vi "refreshRunFolder.vi"(8 "error in (no error)":errorcluster, 11 "Compiler in":refnum<class "Compiler.lvclass">) -> (0 "error out":errorcluster, 3 "Compiler out":refnum<class "Compiler.lvclass">)   [LabVIEW 2009, in "Compiler.lvlib" / "Compiler.lvclass"]
uses:
  Compiler.lvclass
  Compiler.lvclass/Compiler.ctl
  Filing/FileSystem/FileSystem.lvclass
panel:
  # "database has changed\nso all scripts should be\nrecompiled"
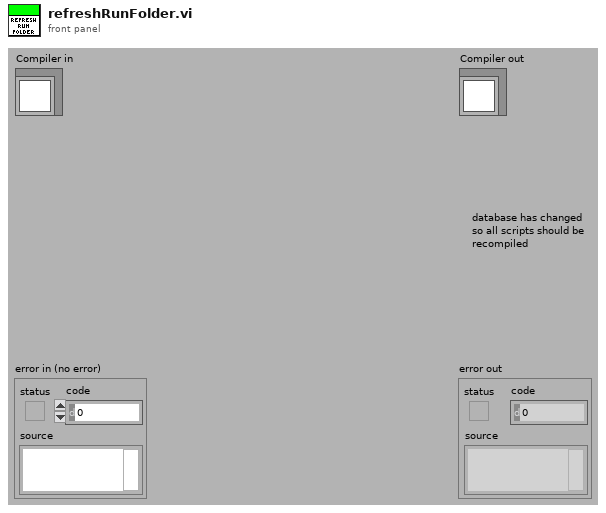
[diagram p1: front panel]
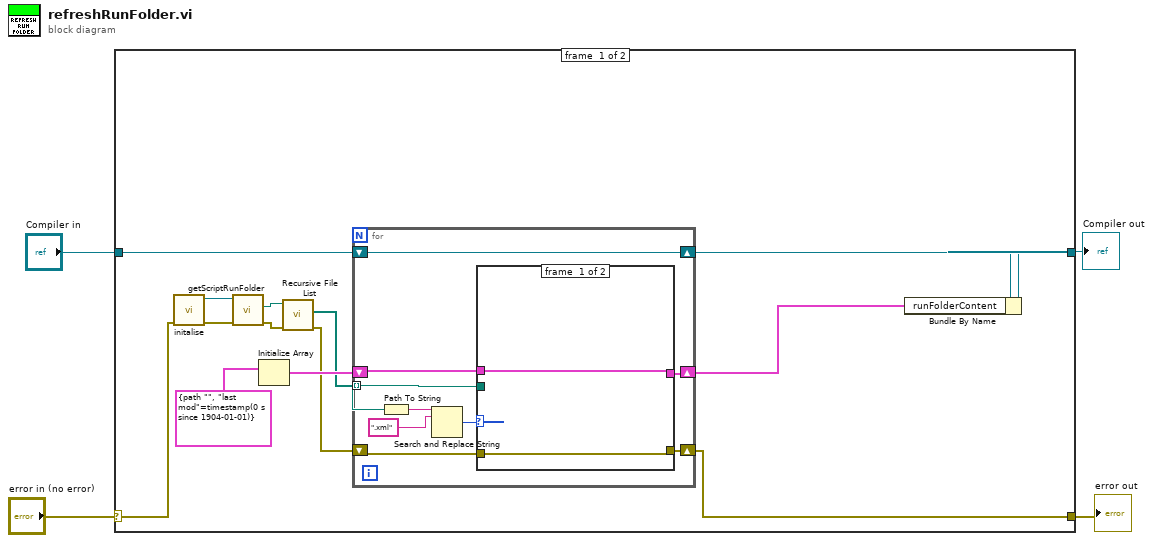
[diagram p0: block diagram]
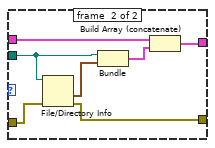
[diagram p2: hidden frame]
diagram:
  n1 = case shown="No Error" "error in (no error)" {
    selector: "error in (no error)" -> [w14 w38]
    tunnel: [w5 w38] -> w3
    tunnel: [w11 w37] -> w1
    tunnel: "Compiler in" -> [w9 w37]
    frame #0 {
      n2 = call "initalise.vi"("error in (no error)"=w14) -> ("error out"=w17:errorcluster, "FileSystem out"=w18:refnum<class "FileSystem.lvclass">)  [unwired: 9 in]
      n3 = call "getScriptRunFolder.vi"("error in (no error)"=w17, "FileSystem.lvclass in"=w18) -> ("error out"=w10:errorcluster, "ScriptRunFolder"=w16:path)  [unwired: 7 in, 1 out]
      n4 = Initialize Array(cluster{path, "last mod":timestamp} {path "", "last mod"=timestamp(0 s since 1904-01-01)} ("output cluster")) -> (w15:cluster{path, "last mod":timestamp}[])  [unwired: 1 in]
      n5 = call <vilib>:"Recursive File List.vi"("error in (no error)"=w10, "Folder Path"=w16) -> ("error out"=w6:errorcluster, "All Files in Dir"=w7:path[])  [unwired: 5 in, 3 out]
      n6 = for {
        tunnel: w7 -> [w23] mode=indexing
        shift-right: [w22] -> w8
        shift-left: w15 -> [w24]
        shift-right: [w21] -> w12
        shift-left: w9 -> [w21]
        shift-right: [w19] -> w5
        shift-left: w6 -> [w20]
        n7 = Path To String(path=w23) -> (string=w27:string)
        n8 = Search and Replace String(input string=w27, search string=".xml") -> (number of replacements=w25:i32)  [unwired: 6 in, 3 out]
        n9 = case shown="1, Default" w25 {
          tunnel: w24 -> [w29 w34]
          tunnel: w23 -> [_ w36]
          tunnel: [w29 w32] -> w22
          tunnel: w20 -> [w28 w31]
          tunnel: [w28 w30] -> w19
          frame #0 {
          }
          frame #1 {
            n10 = File/Directory Info(path=w36, error in=w31) -> (last mod=w35:timestamp, error out=w30:errorcluster)  [unwired: 5 out]
            n11 = Bundle(w36, "last mod"=w35) -> (w33:cluster{path, "last mod":timestamp})  [unwired: 1 in]
            n12 = Build Array (concatenate)(w34, w33) -> (w32:cluster{path, "last mod":timestamp}[])
          }
        }
      }
      n13 = Bundle By Name(cluster=w12, "runFolderContent"=w8) -> (w11:refnum<class "Compiler.lvclass">)
    }
    frame #1 {
    }
  }
  "error out" <- w3
  "Compiler out" <- w1
